vi "函数类型1测试.vi"() -> ()   [LabVIEW 2010]
uses:
  全局量/试验配置信息.vi
panel:
  out "D_IN_1":string[][](table) caption="表格"
  in  "加载文件名称":string
  out "配置文件路径":path
  out "配置文件目录":path
  in  "同步_1":i32
  in  "数组_反馈值":dbl[][](array[numeric])
  in  "第几个数据":i32
  in  "第几组数据":i32
  in  "数组_设定值":dbl[][](array[numeric])
  in  "数组_选择":bool[](array[boolean])
  out "light_32":bool
  out "light_31":bool
  out "light_30":bool
  out "light_29":bool
  out "light_28":bool
  out "light_27":bool
  out "light_26":bool
  out "light_25":bool
  out "light_24":bool
  out "light_23":bool
  out "light_22":bool
  out "light_21":bool
  out "light_20":bool
  out "light_19":bool
  out "light_18":bool
  out "light_17":bool
  out "Analog_back":string[][](table) caption="表格"
  in  "A_32":bool
  in  "A_31":bool
  in  "A_30":bool
  in  "A_29":bool
  in  "A_28":bool
  in  "A_27":bool
  in  "A_26":bool
  in  "A_25":bool
  in  "A_24":bool
  in  "A_23":bool
  in  "A_22":bool
  in  "A_21":bool
  in  "A_20":bool
  in  "A_19":bool
  in  "A_18":bool
  in  "A_17":bool
  out "合格？":bool[][](array[boolean])
  out "测试结论":string
  out "light_16":bool
  out "light_15":bool
  out "light_14":bool
  out "light_13":bool
  out "light_12":bool
  out "light_11":bool
  out "light_10":bool
  out "light_9":bool
  out "light_8":bool
  out "light_7":bool
  out "light_6":bool
  out "light_5":bool
  out "light_4":bool
  out "light_3":bool
  out "light_2":bool
  out "light_1":bool
  out "退出？":bool
  in  "btn_反选":bool
  in  "btn_全选":bool
  in  "A_16":bool
  in  "A_15":bool
  in  "A_14":bool
  in  "A_13":bool
  in  "A_12":bool
  in  "A_11":bool
  in  "A_10":bool
  in  "A_9":bool
  in  "A_8":bool
  in  "A_7":bool
  in  "A_6":bool
  in  "A_5":bool
  in  "A_4":bool
  in  "A_3":bool
  in  "A_2":bool
  in  "A_1":bool
  in  "btn_取消":bool
  in  "btn_开始测试":bool
  in  "Analog_IN":string[][](table) caption="表格"
  out "Analog_WC":string[][](table) caption="表格"
  # "模拟量选择及输入值（V）"
  # "模拟量反馈值（V）"
  # "模拟量误差值（%）"
  # "测试结论："
  # "从0开始"
  # "从1开始,第0列没有使用"
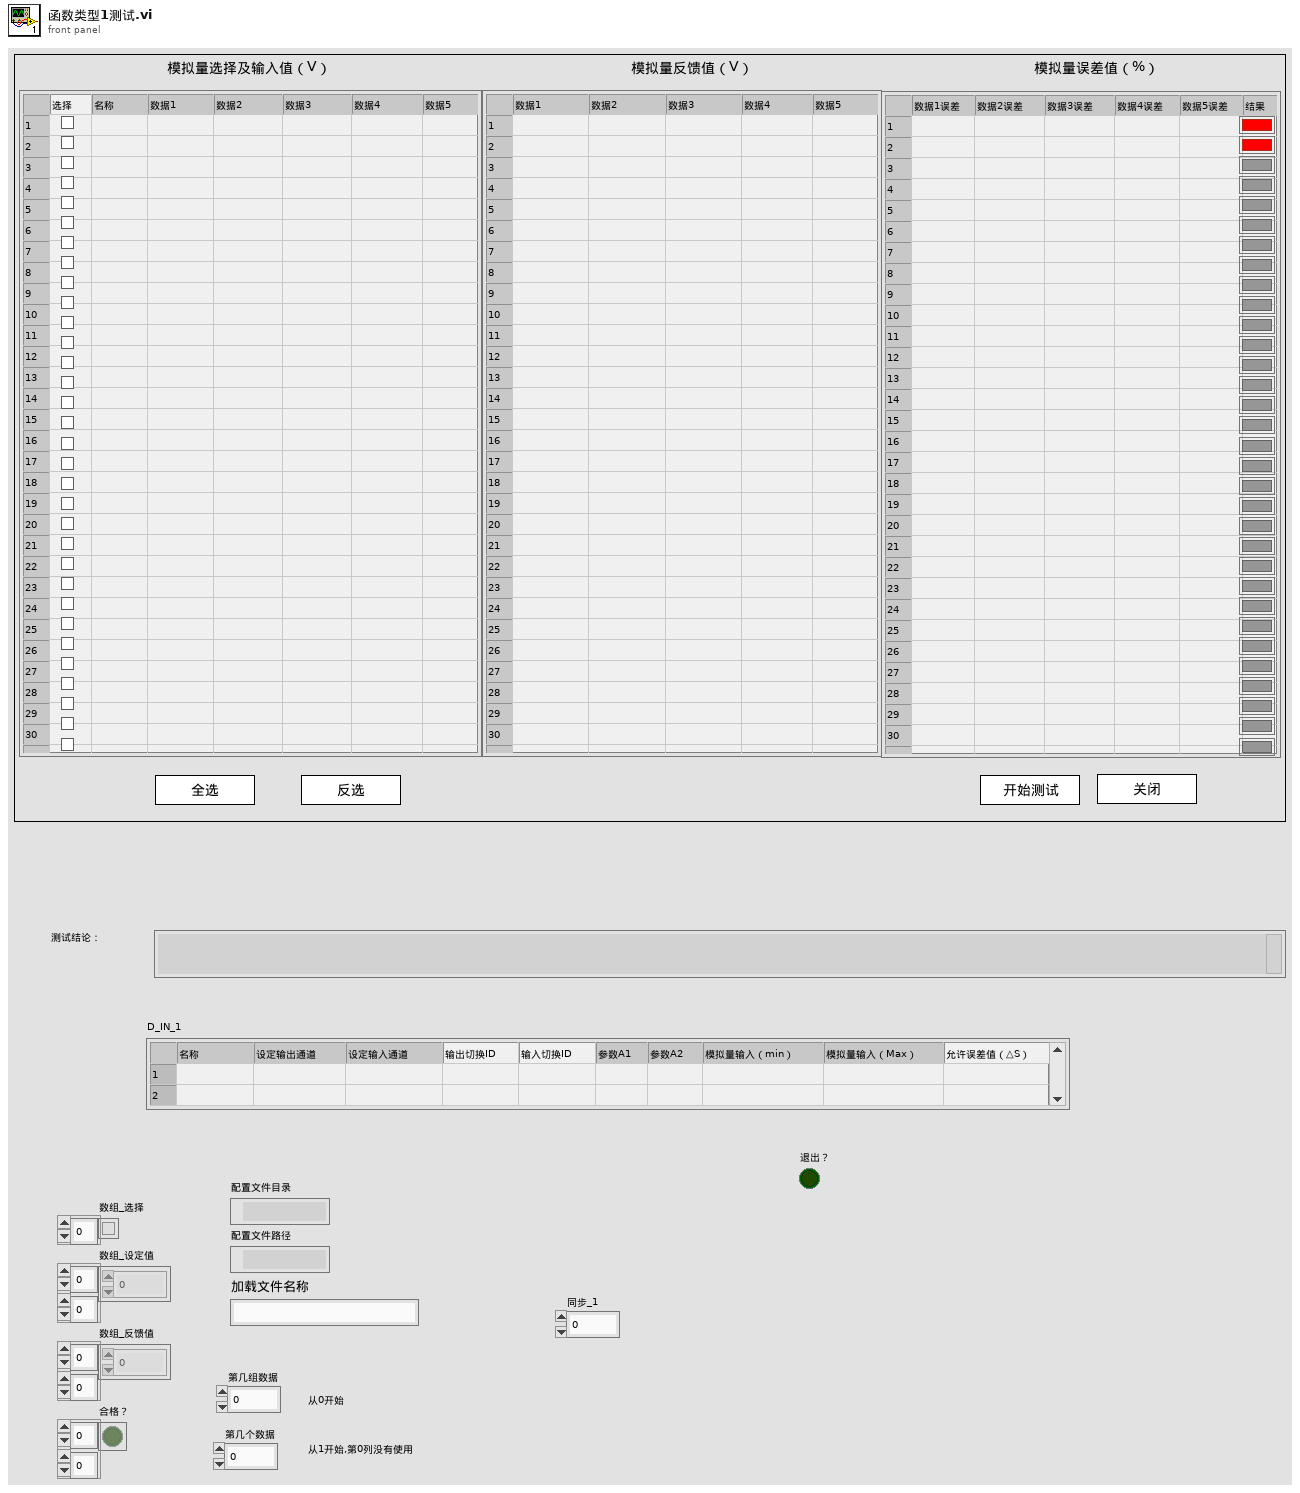
[diagram p1: front panel]
types:
  T1 = enum8{"Enabled", "Disabled", "Disabled and Grayed Out"}
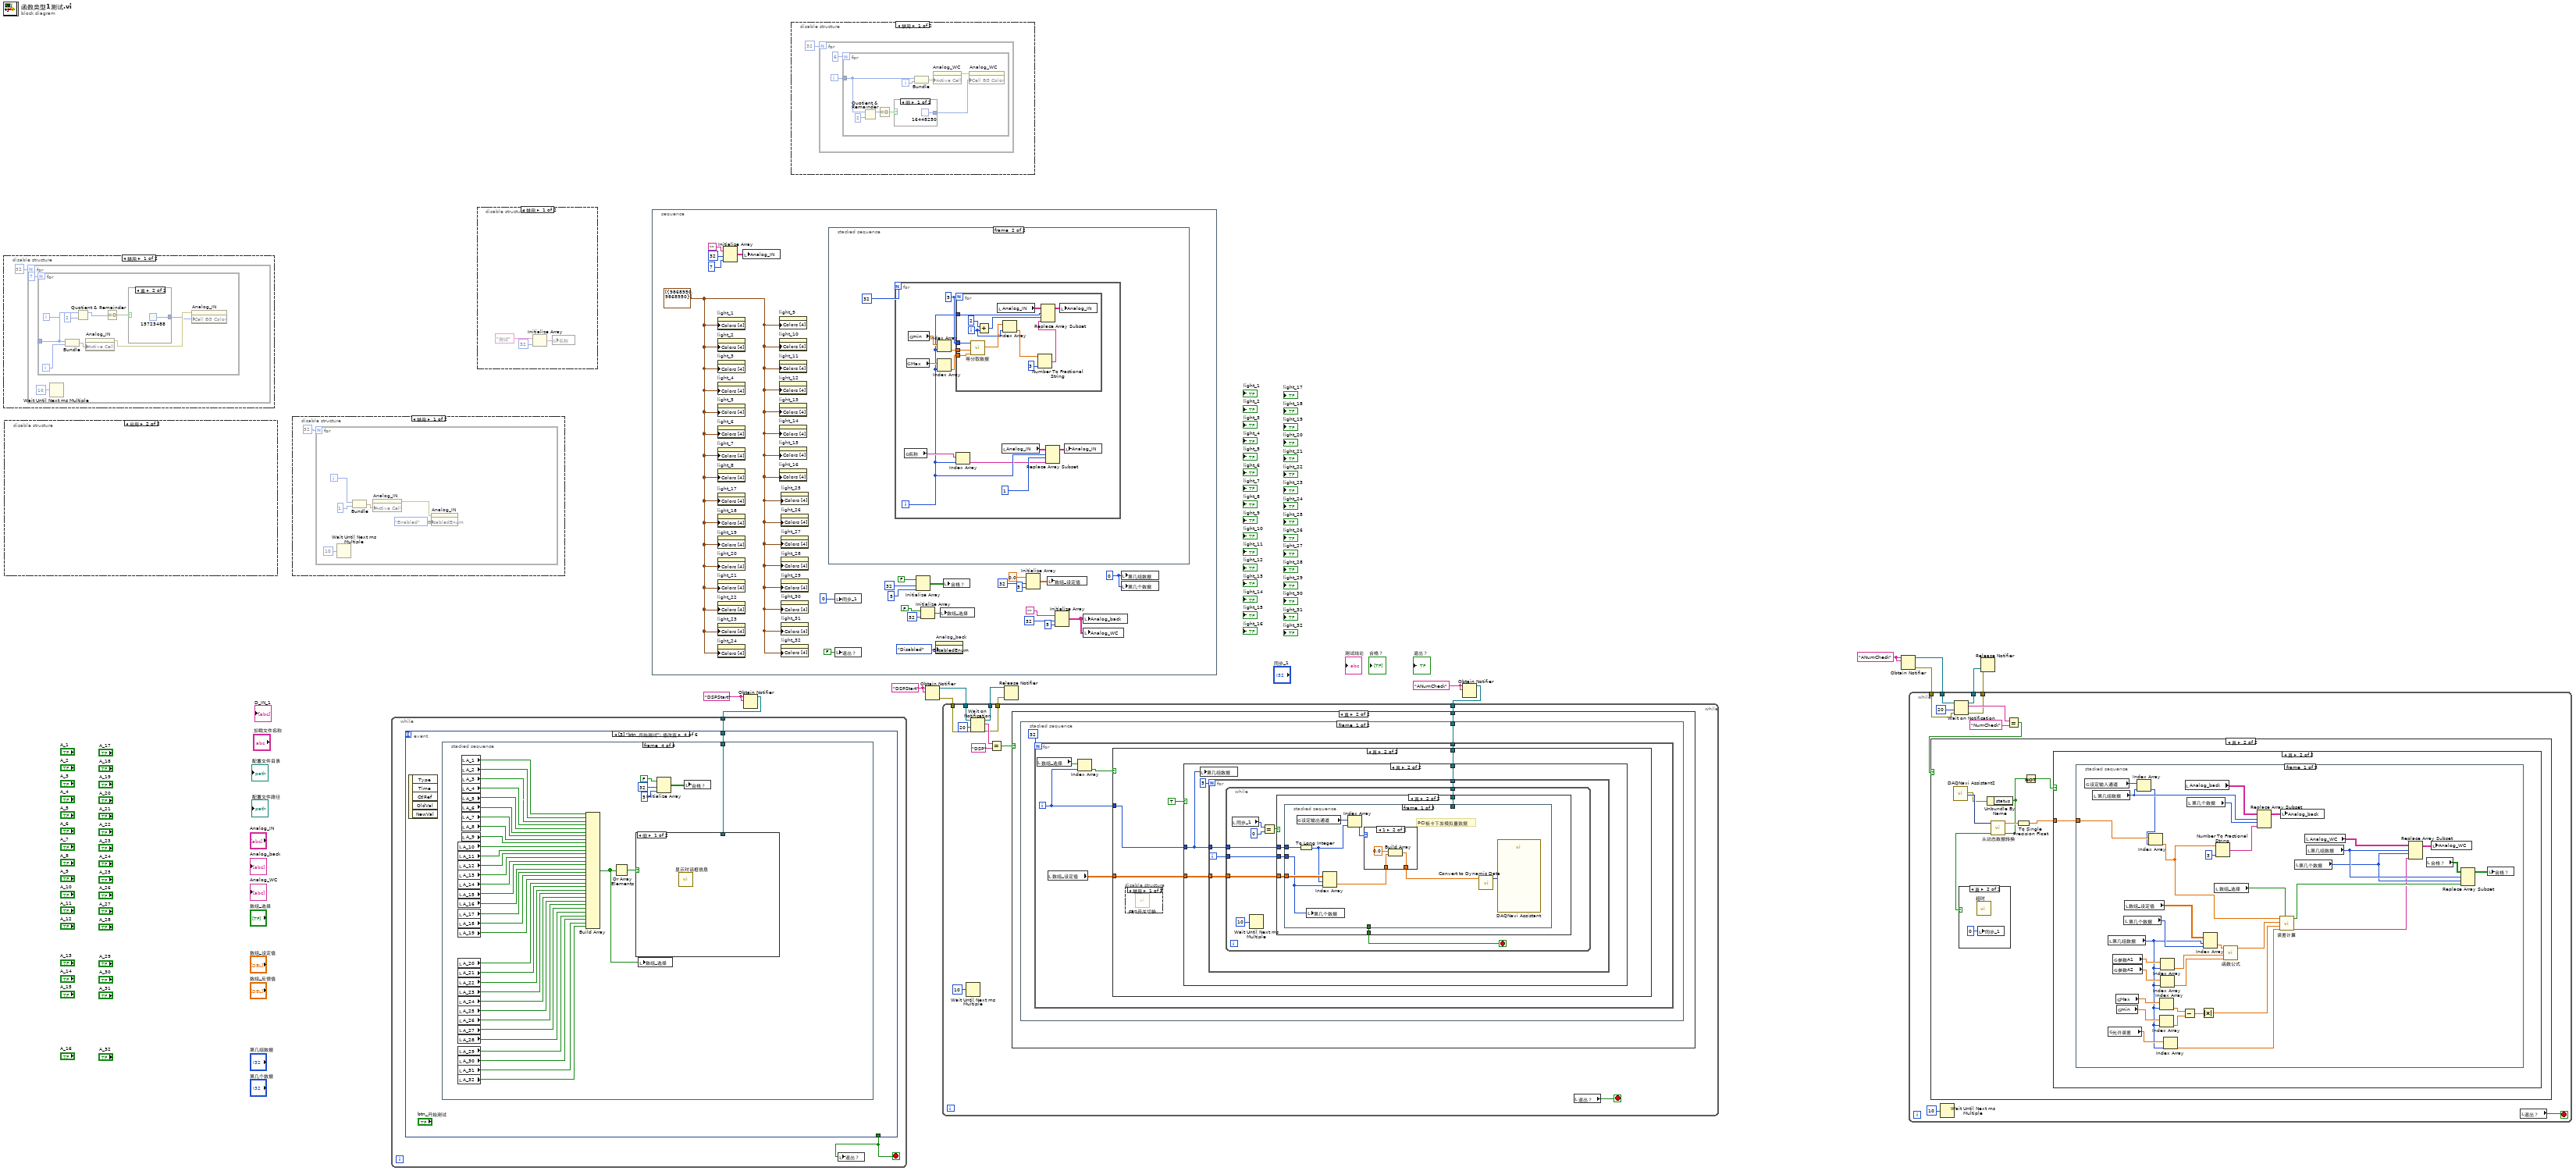
[diagram p0: block diagram]
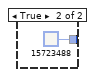
[diagram p2: hidden frame]
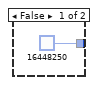
[diagram p5: hidden frame]
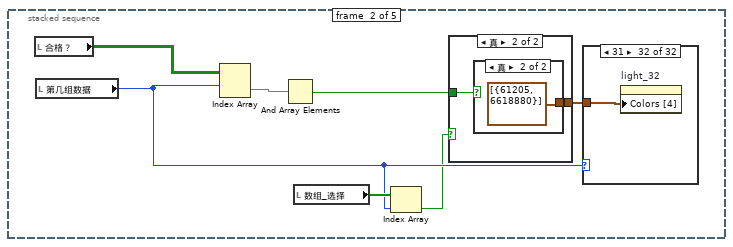
[diagram p10: hidden frame]
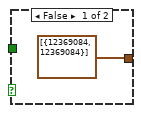
[diagram p11: hidden frame]
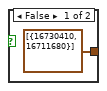
[diagram p12: hidden frame]
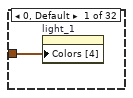
[diagram p13: hidden frame]
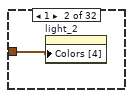
[diagram p14: hidden frame]
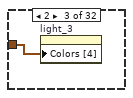
[diagram p15: hidden frame]
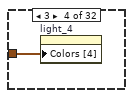
[diagram p16: hidden frame]
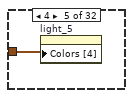
[diagram p17: hidden frame]
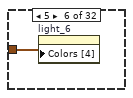
[diagram p18: hidden frame]
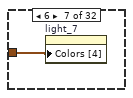
[diagram p19: hidden frame]
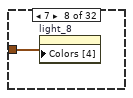
[diagram p20: hidden frame]
diagram:
  w2 = "ANumCheck" ("名称（未命名）")
  w4 = "DSPStart" ("名称（未命名）")
  w9 = "ANumCheck" ("名称（未命名）")
  w12 = "DSPStart" ("名称（未命名）")
  n1 = disable-structure shown="禁用" {
    frame Disabled {
      n2 = for {
        N: 32 -> [_]
        i -> [w17]
        n3 = for {
          N: 7 -> [_]
          tunnel: w17 -> [w25]
          i -> [w19]
          n4 = Bundle(w25, w19) -> (w22:cluster{i32, i32})  [unwired: 1 in]
          n5 = Quotient & Remainder(x=w25, y=2) -> (x-y*floor(x/y)=w23:i32)  [unwired: 1 out]
          n6 = property on="Analog_IN" class="Tbl (严格)"("Active Cell"=w22) -> (error out=w21:errorcluster)  [unwired: 2 in, 1 out]
          n7 = Equal To 0?(x=w23) -> (x = 0?=w26:bool)
          n8 = case shown="真" w26 {
            tunnel: [u32 16448250 u32 15723488] -> w20
            frame False {
            }
            frame True {
            }
          }
          n9 = property on="Analog_IN" class="Tbl (严格)"(error in=w21, "Cell BG Color"=w20) -> ()  [unwired: 1 in, 2 out]
        }
        n10 = Wait Until Next ms Multiple(millisecond multiple=u32 10 ("毫秒倍数")) -> ()  [unwired: 1 out]
      }
    }
    frame Enabled {
    }
  }
  n11 = disable-structure shown="启用" {
    frame Disabled {
      n12 = for {
        N: 32 -> [_]
        i -> [w30]
        n13 = for {
          N: 7 -> [_]
          tunnel: w30 -> [w33]
          i -> [w34]
          n14 = Bundle(w33, w34) -> (w37:cluster{i32, i32})  [unwired: 1 in]
          n15 = property on="Analog_IN" class="Tbl (严格)"("Active Cell"=w37) -> (error out=w35:errorcluster)  [unwired: 2 in, 1 out]
          n16 = property on="Analog_IN" class="Tbl (严格)"(error in=w35, "Justify"=enum16{"Left", "Center", "Right"}."Left" ("活动单元格:单元格对齐")) -> ()  [unwired: 1 in, 2 out]
        }
        n17 = Wait Until Next ms Multiple(millisecond multiple=u32 10 ("毫秒倍数")) -> ()  [unwired: 1 out]
      }
    }
    frame Enabled {
    }
  }
  n18 = disable-structure shown="禁用" {
    frame Disabled {
      n19 = for {
        N: 32 -> [_]
        i -> [w43]
        n20 = Wait Until Next ms Multiple(millisecond multiple=u32 10 ("毫秒倍数")) -> ()  [unwired: 1 out]
        n21 = Bundle(w43, 1) -> (w42:cluster{i32, i32})  [unwired: 1 in]
        n22 = property on="Analog_IN" class="Tbl (严格)"("Active Cell"=w42) -> (error out=w39:errorcluster)  [unwired: 2 in, 1 out]
        n23 = property on="Analog_IN" class="Tbl (严格)"(error in=w39, "DisabledEnum"=T1."Enabled" ("禁用")) -> ()  [unwired: 1 in, 2 out]
      }
    }
    frame Enabled {
    }
  }
  n24 = disable-structure shown="禁用" {
    frame Disabled {
      n25 = Initialize Array("测试", 32 ("维数大小")) -> (w46:string[])
      n26 = global write "试验配置信息.vi" "名称"(w46) -> ()
    }
    frame Enabled {
    }
  }
  n27 = stacked-sequence {
    frame #0 {
      w52 = 0 ("第几组数据")
      w67 = cluster{u32, u32}[] [{9868950, 9868950}]
      n28 = property on="light_1" class="Bool (严格)"("Colors [4]"=w67) -> ()  [unwired: 2 in, 2 out]
      n29 = property on="light_2" class="Bool (严格)"("Colors [4]"=w67) -> ()  [unwired: 2 in, 2 out]
      n30 = property on="light_3" class="Bool (严格)"("Colors [4]"=w67) -> ()  [unwired: 2 in, 2 out]
      n31 = property on="light_4" class="Bool (严格)"("Colors [4]"=w67) -> ()  [unwired: 2 in, 2 out]
      n32 = property on="light_5" class="Bool (严格)"("Colors [4]"=w67) -> ()  [unwired: 2 in, 2 out]
      n33 = property on="light_6" class="Bool (严格)"("Colors [4]"=w67) -> ()  [unwired: 2 in, 2 out]
      n34 = property on="light_7" class="Bool (严格)"("Colors [4]"=w67) -> ()  [unwired: 2 in, 2 out]
      n35 = property on="light_8" class="Bool (严格)"("Colors [4]"=w67) -> ()  [unwired: 2 in, 2 out]
      n36 = property on="light_17" class="Bool (严格)"("Colors [4]"=w67) -> ()  [unwired: 2 in, 2 out]
      n37 = property on="light_18" class="Bool (严格)"("Colors [4]"=w67) -> ()  [unwired: 2 in, 2 out]
      n38 = property on="light_19" class="Bool (严格)"("Colors [4]"=w67) -> ()  [unwired: 2 in, 2 out]
      n39 = property on="light_20" class="Bool (严格)"("Colors [4]"=w67) -> ()  [unwired: 2 in, 2 out]
      n40 = property on="light_21" class="Bool (严格)"("Colors [4]"=w67) -> ()  [unwired: 2 in, 2 out]
      n41 = property on="light_22" class="Bool (严格)"("Colors [4]"=w67) -> ()  [unwired: 2 in, 2 out]
      n42 = property on="light_23" class="Bool (严格)"("Colors [4]"=w67) -> ()  [unwired: 2 in, 2 out]
      n43 = property on="light_24" class="Bool (严格)"("Colors [4]"=w67) -> ()  [unwired: 2 in, 2 out]
      n44 = Initialize Array("", 32 ("维数大小"), 7 ("维数大小")) -> (w51:string[][])
      n45 = local write "Analog_IN"(w51) -> ()
      n46 = property on="light_9" class="Bool (严格)"("Colors [4]"=w67) -> ()  [unwired: 2 in, 2 out]
      n47 = property on="light_10" class="Bool (严格)"("Colors [4]"=w67) -> ()  [unwired: 2 in, 2 out]
      n48 = property on="light_11" class="Bool (严格)"("Colors [4]"=w67) -> ()  [unwired: 2 in, 2 out]
      n49 = property on="light_12" class="Bool (严格)"("Colors [4]"=w67) -> ()  [unwired: 2 in, 2 out]
      n50 = property on="light_13" class="Bool (严格)"("Colors [4]"=w67) -> ()  [unwired: 2 in, 2 out]
      n51 = property on="light_14" class="Bool (严格)"("Colors [4]"=w67) -> ()  [unwired: 2 in, 2 out]
      n52 = property on="light_15" class="Bool (严格)"("Colors [4]"=w67) -> ()  [unwired: 2 in, 2 out]
      n53 = property on="light_16" class="Bool (严格)"("Colors [4]"=w67) -> ()  [unwired: 2 in, 2 out]
      n54 = property on="light_25" class="Bool (严格)"("Colors [4]"=w67) -> ()  [unwired: 2 in, 2 out]
      n55 = property on="light_26" class="Bool (严格)"("Colors [4]"=w67) -> ()  [unwired: 2 in, 2 out]
      n56 = property on="light_27" class="Bool (严格)"("Colors [4]"=w67) -> ()  [unwired: 2 in, 2 out]
      n57 = property on="light_28" class="Bool (严格)"("Colors [4]"=w67) -> ()  [unwired: 2 in, 2 out]
      n58 = property on="light_29" class="Bool (严格)"("Colors [4]"=w67) -> ()  [unwired: 2 in, 2 out]
      n59 = property on="light_30" class="Bool (严格)"("Colors [4]"=w67) -> ()  [unwired: 2 in, 2 out]
      n60 = property on="light_31" class="Bool (严格)"("Colors [4]"=w67) -> ()  [unwired: 2 in, 2 out]
      n61 = property on="light_32" class="Bool (严格)"("Colors [4]"=w67) -> ()  [unwired: 2 in, 2 out]
      n62 = stacked-sequence {
        frame #0 {
          n63 = for {
            N: 32 ("维数大小") -> [_]
            tunnel: [w112] -> w76 mode=indexing
            tunnel: [w108] -> w75 mode=indexing
            tunnel: [w106] -> w74 mode=indexing
            tunnel: [w103] -> w73 mode=indexing
            tunnel: [w100] -> w72 mode=indexing
            tunnel: [w97] -> w78 mode=indexing
            tunnel: [w94] -> w79 mode=indexing
            tunnel: [w91] -> w80 mode=indexing
            tunnel: [w88] -> w81 mode=indexing
            tunnel: [w84] -> w82 mode=indexing
            i -> [w86]
            n64 = global read "试验配置信息.vi" "D_IN_1"() -> (w83:string[][])
            n65 = Index Array(array=w83, index (row)=w86, index (col)=0 ("禁用的索引 (列)")) -> (element=w112:string)
            n66 = Index Array(array=w83, index (row)=w86, index (col)=2 ("禁用的索引 (列)")) -> (element=w102:string)
            n67 = Index Array(array=w83, index (row)=w86, index (col)=3 ("禁用的索引 (列)")) -> (element=w98:string)
            n68 = Index Array(array=w83, index (row)=w86, index (col)=4 ("禁用的索引 (列)")) -> (element=w96:string)
            n69 = Index Array(array=w83, index (row)=w86, index (col)=5 ("禁用的索引 (列)")) -> (element=w93:string)
            n70 = Index Array(array=w83, index (row)=w86, index (col)=9 ("禁用的索引 (列)")) -> (element=w85:string)
            n71 = Index Array(array=w83, index (row)=w86, index (col)=1 ("禁用的索引 (列)")) -> (element=w105:string)
            n72 = Index Array(array=w83, index (row)=w86, index (col)=6 ("禁用的索引 (列)")) -> (element=w89:string)
            n73 = Index Array(array=w83, index (row)=w86, index (col)=7 ("禁用的索引 (列)")) -> (element=w109:string)
            n74 = Index Array(array=w83, index (row)=w86, index (col)=8 ("禁用的索引 (列)")) -> (element=w107:string)
            n75 = Decimal String To Number(string=w102) -> (number=w100:i32)  [unwired: 2 in, 1 out]
            n76 = Decimal String To Number(string=w98) -> (number=w97:i32)  [unwired: 2 in, 1 out]
            n77 = Decimal String To Number(string=w96) -> (number=w94:i32)  [unwired: 2 in, 1 out]
            n78 = Decimal String To Number(string=w105) -> (number=w103:i32)  [unwired: 2 in, 1 out]
            n79 = Fract/Exp String To Number(string=w93) -> (number=w91:dbl)  [unwired: 3 in, 1 out]
            n80 = Fract/Exp String To Number(string=w85) -> (number=w84:dbl)  [unwired: 3 in, 1 out]
            n81 = Fract/Exp String To Number(string=w89) -> (number=w88:dbl)  [unwired: 3 in, 1 out]
            n82 = Fract/Exp String To Number(string=w109) -> (number=w108:dbl)  [unwired: 3 in, 1 out]
            n83 = Fract/Exp String To Number(string=w107) -> (number=w106:dbl)  [unwired: 3 in, 1 out]
          }
          n84 = global write "试验配置信息.vi" "名称"(w76) -> ()
          n85 = global write "试验配置信息.vi" "设定输入通道"(w72) -> ()
          n86 = global write "试验配置信息.vi" "输出切换ID"(w78) -> ()
          n87 = global write "试验配置信息.vi" "输入切换ID"(w79) -> ()
          n88 = global write "试验配置信息.vi" "参数A1"(w80) -> ()
          n89 = global write "试验配置信息.vi" "允许误差"(w82) -> ()
          n90 = global write "试验配置信息.vi" "设定输出通道"(w73) -> ()
          n91 = global write "试验配置信息.vi" "参数A2"(w81) -> ()
          n92 = global write "试验配置信息.vi" "min"(w75) -> ()
          n93 = global write "试验配置信息.vi" "Max"(w74) -> ()
        }
        frame #1 {
          n94 = for {
            N: 32 -> [_]
            i -> [w117]
            w121 = 5 ("num")
            n95 = global read "试验配置信息.vi" "名称"() -> (w120:string[])
            n96 = global read "试验配置信息.vi" "Max"() -> (w124:dbl[])
            n97 = global read "试验配置信息.vi" "min"() -> (w125:dbl[])
            n98 = Index Array(array=w125, index=w117) -> (element=w123:dbl)
            n99 = Index Array(array=w124, index=w117) -> (element=w122:dbl)
            n100 = for {
              N: w121 -> [_]
              tunnel: w117 -> [w136]
              tunnel: w123 -> [w133]
              tunnel: w122 -> [w132]
              tunnel: w121 -> [w131]
              i -> [w129]
              n101 = call "等分取数据.vi"("Max"=w132, "MIN"=w133, "num"=w131) -> ("数据点"=w130:dbl[])  [unwired: 5 in]
              n102 = Add(x=2, y=w129) -> (x+y=w134:i32)
              n103 = local read "Analog_IN"() -> (w138:string[][])
              n104 = Index Array(array=w130, index=w129) -> (element=w127:dbl)
              n105 = Number To Fractional String(number=w127, precision (6)=i16 3 ("精度(6)")) -> (F-format string=w128:string)  [unwired: 2 in]
              n106 = Replace Array Subset(array=w138, new element=w128, index (row)=w136, index (col)=w134) -> (w137:string[][])
              n107 = local write "Analog_IN"(w137) -> ()
            }
            n108 = Index Array(array=w120, index=w117) -> (element=w115:string)
            n109 = local read "Analog_IN"() -> (w118:string[][])
            n110 = Replace Array Subset(array=w118, new element=w115, index (row)=w117, index (col)=1) -> (w119:string[][])
            n111 = local write "Analog_IN"(w119) -> ()
          }
        }
      }
      n112 = local write "同步_1"(0 ("同步_2")) -> ()
      n113 = local write "退出？"(FALSE ("退出？")) -> ()
      n114 = Initialize Array(FALSE, 32 ("维数大小"), 5 ("维数大小")) -> (w68:bool[][])
      n115 = Initialize Array(FALSE, 32 ("维数大小")) -> (w56:bool[])
      n116 = property on="Analog_back" class="Tbl (严格)"("DisabledEnum"=T1."Disabled" ("禁用")) -> ()  [unwired: 2 in, 2 out]
      n117 = local write "数组_选择"(w56) -> ()
      n118 = local write "合格？"(w68) -> ()
      n119 = Initialize Array(0.0, 32 ("维数大小"), 5 ("维数大小")) -> (w59:dbl[][])
      n120 = local write "数组_设定值"(w59) -> ()
      n121 = Initialize Array("", 32 ("维数大小"), 5 ("维数大小")) -> (w63:string[][])
      n122 = local write "Analog_back"(w63) -> ()
      n123 = local write "Analog_WC"(w63) -> ()
      n124 = local write "第几组数据"(w52) -> ()
      n125 = local write "第几个数据"(w52) -> ()
    }
  }
  n126 = Obtain Notifier(name (unnamed)=w4, notification data type=w4) -> (notifier out=w3:refnum<notifier>)  [unwired: 2 in, 2 out]
  n127 = while {
    tunnel: w3 -> [w139]
    stop <- w140 stop-if-true
    n128 = event shown="[3] \"btn_开始测试\": 值改变" {
      selector: _ -> [_ _ _ _ _ _]
      dyn-events: _ -> [_ _ _ _ _ _]
      timeout: _ -> [_ _ _ _ _ _]
      tunnel: [_ TRUE TRUE _ _ _] -> w140
      tunnel: w139 -> [_ _ _ w143 _ _]
      event Timeout {
        n129 = event-data() -> ()  [unwired: 1 in, 2 out]
      }
      event Panel Close {
        n130 = event-data() -> ()  [unwired: 1 in, 3 out]
      }
      event "btn_取消": Value Change {
        n131 = event-data() -> ()  [unwired: 1 in, 5 out]
      }
      event "btn_开始测试": Value Change {
        n132 = event-data() -> ()  [unwired: 1 in, 5 out]
        n133 = stacked-sequence {
          tunnel: w143 -> [_ _ _ w226]
          frame #0 {
            w149 = 0 ("第几组数据")
            # "测试期间不准退出防止程序卡死"
            n134 = local read "Analog_IN"() -> (w155:string[][])
            n135 = Delete From Array(array=w155, length=1 ("长度"), index (col)=0 ("禁用的索引 (列)")) -> (array with subset deleted=w147:string[][])  [unwired: 1 in, 1 out]
            n136 = Delete From Array(array=w147, length=1 ("长度"), index (col)=0 ("禁用的索引 (列)")) -> (array with subset deleted=w145:string[][])  [unwired: 1 in, 1 out]
            n137 = for {
              N: 32 -> [_]
              tunnel: w145 -> [w158] mode=indexing
              tunnel: [w157] -> w154 mode=indexing
              n138 = for {
                N: 5 -> [_]
                tunnel: w158 -> [w160] mode=indexing
                tunnel: [w159] -> w157 mode=indexing
                n139 = Fract/Exp String To Number(string=w160) -> (number=w159:dbl)  [unwired: 3 in, 1 out]
              }
            }
            n140 = local write "第几组数据"(w149) -> ()
            n141 = local write "第几个数据"(w149) -> ()
            n142 = local write "同步_1"(0 ("同步_2")) -> ()
            n143 = property on="btn_取消" class="Bool"("DisabledEnum"=T1."Disabled and Grayed Out" ("禁用")) -> ()  [unwired: 2 in, 2 out]
            n144 = local write "数组_设定值"(w154) -> ()
          }
          frame #1 {
            n145 = local read "Analog_back"() -> (w163:string[][])
            n146 = local read "Analog_WC"() -> (w162:string[][])
            n147 = for {
              tunnel: w162 -> [w199] mode=indexing
              i -> [w198]
              n148 = for {
                tunnel: w199 -> [_] mode=indexing
                tunnel: w198 -> [w203]
                i -> [w202]
                n149 = local read "Analog_WC"() -> (w204:string[][])
                n150 = Replace Array Subset(array=w204, new element="", index (row)=w203, index (col)=w202) -> (w200:string[][])
                n151 = local write "Analog_WC"(w200) -> ()
              }
            }
            n152 = for {
              tunnel: w163 -> [w206] mode=indexing
              i -> [w205]
              n153 = for {
                tunnel: w206 -> [_] mode=indexing
                tunnel: w205 -> [w210]
                i -> [w209]
                n154 = local read "Analog_back"() -> (w211:string[][])
                n155 = Replace Array Subset(array=w211, new element="", index (row)=w210, index (col)=w209) -> (w207:string[][])
                n156 = local write "Analog_back"(w207) -> ()
              }
            }
            n157 = for {
              N: 32 -> [_]
              i -> [w165]
              n158 = case shown="31" w165 {
                tunnel: cluster{u32, u32}[] [{9868950, 9868950}] -> [w166 w167 w168 w169 w170 w171 w172 w173 w174 w175 w176 w177 w178 w179 w180 w181 w182 w183 w184 w185 w186 w187 w188 w189 w190 w191 w192 w193 w194 w195 w196 w197]
                frame 0, Default {
                  n159 = property on="light_1" class="Bool (严格)"("Colors [4]"=w166) -> ()  [unwired: 2 in, 2 out]
                }
                frame 1 {
                  n160 = property on="light_2" class="Bool (严格)"("Colors [4]"=w167) -> ()  [unwired: 2 in, 2 out]
                }
                frame 2 {
                  n161 = property on="light_3" class="Bool (严格)"("Colors [4]"=w168) -> ()  [unwired: 2 in, 2 out]
                }
                frame 3 {
                  n162 = property on="light_4" class="Bool (严格)"("Colors [4]"=w169) -> ()  [unwired: 2 in, 2 out]
                }
                frame 4 {
                  n163 = property on="light_5" class="Bool (严格)"("Colors [4]"=w170) -> ()  [unwired: 2 in, 2 out]
                }
                frame 5 {
                  n164 = property on="light_6" class="Bool (严格)"("Colors [4]"=w171) -> ()  [unwired: 2 in, 2 out]
                }
                frame 6 {
                  n165 = property on="light_7" class="Bool (严格)"("Colors [4]"=w172) -> ()  [unwired: 2 in, 2 out]
                }
                frame 7 {
                  n166 = property on="light_8" class="Bool (严格)"("Colors [4]"=w173) -> ()  [unwired: 2 in, 2 out]
                }
                frame 8 {
                  n167 = property on="light_9" class="Bool (严格)"("Colors [4]"=w174) -> ()  [unwired: 2 in, 2 out]
                }
                frame 9 {
                  n168 = property on="light_10" class="Bool (严格)"("Colors [4]"=w175) -> ()  [unwired: 2 in, 2 out]
                }
                frame 10 {
                  n169 = property on="light_11" class="Bool (严格)"("Colors [4]"=w176) -> ()  [unwired: 2 in, 2 out]
                }
                frame 11 {
                  n170 = property on="light_12" class="Bool (严格)"("Colors [4]"=w177) -> ()  [unwired: 2 in, 2 out]
                }
                frame 12 {
                  n171 = property on="light_13" class="Bool (严格)"("Colors [4]"=w178) -> ()  [unwired: 2 in, 2 out]
                }
                frame 13 {
                  n172 = property on="light_14" class="Bool (严格)"("Colors [4]"=w179) -> ()  [unwired: 2 in, 2 out]
                }
                frame 14 {
                  n173 = property on="light_15" class="Bool (严格)"("Colors [4]"=w180) -> ()  [unwired: 2 in, 2 out]
                }
                frame 15 {
                  n174 = property on="light_16" class="Bool (严格)"("Colors [4]"=w181) -> ()  [unwired: 2 in, 2 out]
                }
                frame 16 {
                  n175 = property on="light_17" class="Bool (严格)"("Colors [4]"=w182) -> ()  [unwired: 2 in, 2 out]
                }
                frame 17 {
                  n176 = property on="light_18" class="Bool (严格)"("Colors [4]"=w183) -> ()  [unwired: 2 in, 2 out]
                }
                frame 18 {
                  n177 = property on="light_19" class="Bool (严格)"("Colors [4]"=w184) -> ()  [unwired: 2 in, 2 out]
                }
                frame 19 {
                  n178 = property on="light_20" class="Bool (严格)"("Colors [4]"=w185) -> ()  [unwired: 2 in, 2 out]
                }
                frame 20 {
                  n179 = property on="light_21" class="Bool (严格)"("Colors [4]"=w186) -> ()  [unwired: 2 in, 2 out]
                }
                frame 21 {
                  n180 = property on="light_22" class="Bool (严格)"("Colors [4]"=w187) -> ()  [unwired: 2 in, 2 out]
                }
                frame 22 {
                  n181 = property on="light_23" class="Bool (严格)"("Colors [4]"=w188) -> ()  [unwired: 2 in, 2 out]
                }
                frame 23 {
                  n182 = property on="light_24" class="Bool (严格)"("Colors [4]"=w189) -> ()  [unwired: 2 in, 2 out]
                }
                frame 24 {
                  n183 = property on="light_25" class="Bool (严格)"("Colors [4]"=w190) -> ()  [unwired: 2 in, 2 out]
                }
                frame 25 {
                  n184 = property on="light_26" class="Bool (严格)"("Colors [4]"=w191) -> ()  [unwired: 2 in, 2 out]
                }
                frame 26 {
                  n185 = property on="light_27" class="Bool (严格)"("Colors [4]"=w192) -> ()  [unwired: 2 in, 2 out]
                }
                frame 27 {
                  n186 = property on="light_28" class="Bool (严格)"("Colors [4]"=w193) -> ()  [unwired: 2 in, 2 out]
                }
                frame 28 {
                  n187 = property on="light_29" class="Bool (严格)"("Colors [4]"=w194) -> ()  [unwired: 2 in, 2 out]
                }
                frame 29 {
                  n188 = property on="light_30" class="Bool (严格)"("Colors [4]"=w195) -> ()  [unwired: 2 in, 2 out]
                }
                frame 30 {
                  n189 = property on="light_31" class="Bool (严格)"("Colors [4]"=w196) -> ()  [unwired: 2 in, 2 out]
                }
                frame 31 {
                  n190 = property on="light_32" class="Bool (严格)"("Colors [4]"=w197) -> ()  [unwired: 2 in, 2 out]
                }
              }
            }
          }
          frame #2 {
            n191 = for {
              N: 32 -> [_]
              i -> [w214]
              n192 = disable-structure shown="禁用" {
                frame Disabled {
                  n193 = Wait Until Next ms Multiple(millisecond multiple=u32 10 ("毫秒倍数")) -> ()  [unwired: 1 out]
                }
                frame Enabled {
                }
              }
              n194 = for {
                N: 6 -> [_]
                tunnel: w214 -> [w222]
                i -> [w219]
                n195 = Quotient & Remainder(x=w222, y=2) -> (x-y*floor(x/y)=w220:i32)  [unwired: 1 out]
                n196 = Equal To 0?(x=w220) -> (x = 0?=w223:bool)
                n197 = case shown="假" w223 {
                  tunnel: [u32 16448250 u32 15723488] -> w216
                  frame False {
                  }
                  frame True {
                  }
                }
                n198 = Bundle(w222, w219) -> (w218:cluster{i32, i32})  [unwired: 1 in]
                n199 = property on="Analog_WC" class="Tbl (严格)"("Active Cell"=w218) -> (error out=w217:errorcluster)  [unwired: 2 in, 1 out]
                n200 = property on="Analog_WC" class="Tbl (严格)"(error in=w217, "Cell BG Color"=w216) -> ()  [unwired: 1 in, 2 out]
              }
            }
          }
          frame #3 {
            n201 = local read "A_10"() -> (w255:bool)
            n202 = local read "A_11"() -> (w254:bool)
            n203 = local read "A_12"() -> (w253:bool)
            n204 = local read "A_13"() -> (w252:bool)
            n205 = local read "A_14"() -> (w251:bool)
            n206 = local read "A_15"() -> (w250:bool)
            n207 = local read "A_16"() -> (w249:bool)
            n208 = local read "A_17"() -> (w248:bool)
            n209 = local read "A_18"() -> (w247:bool)
            n210 = local read "A_19"() -> (w246:bool)
            n211 = local read "A_20"() -> (w245:bool)
            n212 = local read "A_21"() -> (w244:bool)
            n213 = local read "A_22"() -> (w243:bool)
            n214 = local read "A_23"() -> (w242:bool)
            n215 = local read "A_24"() -> (w241:bool)
            n216 = local read "A_25"() -> (w240:bool)
            n217 = local read "A_26"() -> (w239:bool)
            n218 = local read "A_27"() -> (w238:bool)
            n219 = local read "A_28"() -> (w237:bool)
            n220 = local read "A_29"() -> (w236:bool)
            n221 = local read "A_30"() -> (w235:bool)
            n222 = local read "A_31"() -> (w234:bool)
            n223 = local read "A_32"() -> (w233:bool)
            n224 = local read "A_1"() -> (w264:bool)
            n225 = local read "A_2"() -> (w263:bool)
            n226 = local read "A_3"() -> (w262:bool)
            n227 = local read "A_4"() -> (w261:bool)
            n228 = local read "A_5"() -> (w260:bool)
            n229 = local read "A_6"() -> (w259:bool)
            n230 = local read "A_7"() -> (w258:bool)
            n231 = local read "A_8"() -> (w257:bool)
            n232 = local read "A_9"() -> (w256:bool)
            n233 = Build Array(w264, w263, w262, w261, w260, w259, w258, w257, w256, w255, w254, w253, w252, w251, w250, w249, w248, w247, w246, w245, w244, w243, w242, w241, w240, w239, w238, w237, w236, w235, w234, w233) -> (w227:bool[])
            n234 = Or Array Elements(Boolean array=w227) -> (logical OR=w232:bool)
            n235 = case shown="假" w232 {
              tunnel: w226 -> [_ w265]
              frame False {
                n236 = call "显示对话框信息"() -> ()  [unwired: 10 in, 2 out]
              }
              frame True {
                n237 = Send Notification(notification="DSP" ("通知"), notifier=w265) -> ()  [unwired: 1 in, 2 out]
              }
            }
            n238 = local write "数组_选择"(w227) -> ()
            n239 = Initialize Array(FALSE, 32 ("维数大小"), 5 ("维数大小")) -> (w228:bool[][])
            n240 = local write "合格？"(w228) -> ()
          }
        }
      }
      event "btn_全选": Value Change {
        w267 = TRUE ("单选_AD_1")
        n241 = event-data() -> ()  [unwired: 1 in, 5 out]
        n242 = local write "A_1"(w267) -> ()
        n243 = local write "A_2"(w267) -> ()
        n244 = local write "A_3"(w267) -> ()
        n245 = local write "A_4"(w267) -> ()
        n246 = local write "A_5"(w267) -> ()
        n247 = local write "A_6"(w267) -> ()
        n248 = local write "A_7"(w267) -> ()
        n249 = local write "A_8"(w267) -> ()
        n250 = local write "A_9"(w267) -> ()
        n251 = local write "A_10"(w267) -> ()
        n252 = local write "A_11"(w267) -> ()
        n253 = local write "A_12"(w267) -> ()
        n254 = local write "A_13"(w267) -> ()
        n255 = local write "A_14"(w267) -> ()
        n256 = local write "A_15"(w267) -> ()
        n257 = local write "A_16"(w267) -> ()
        n258 = local write "A_17"(w267) -> ()
        n259 = local write "A_18"(w267) -> ()
        n260 = local write "A_19"(w267) -> ()
        n261 = local write "A_20"(w267) -> ()
        n262 = local write "A_21"(w267) -> ()
        n263 = local write "A_22"(w267) -> ()
        n264 = local write "A_23"(w267) -> ()
        n265 = local write "A_24"(w267) -> ()
        n266 = local write "A_25"(w267) -> ()
        n267 = local write "A_26"(w267) -> ()
        n268 = local write "A_27"(w267) -> ()
        n269 = local write "A_28"(w267) -> ()
        n270 = local write "A_29"(w267) -> ()
        n271 = local write "A_30"(w267) -> ()
        n272 = local write "A_31"(w267) -> ()
        n273 = local write "A_32"(w267) -> ()
      }
      event "btn_反选": Value Change {
        n274 = event-data() -> ()  [unwired: 1 in, 5 out]
        n275 = local read "A_17"() -> (w299:bool)
        n276 = local read "A_18"() -> (w297:bool)
        n277 = local read "A_19"() -> (w295:bool)
        n278 = local read "A_20"() -> (w293:bool)
        n279 = local read "A_21"() -> (w291:bool)
        n280 = local read "A_22"() -> (w289:bool)
        n281 = local read "A_23"() -> (w287:bool)
        n282 = local read "A_24"() -> (w285:bool)
        n283 = local read "A_25"() -> (w283:bool)
        n284 = local read "A_26"() -> (w281:bool)
        n285 = local read "A_27"() -> (w279:bool)
        n286 = local read "A_28"() -> (w277:bool)
        n287 = local read "A_29"() -> (w275:bool)
        n288 = local read "A_30"() -> (w273:bool)
        n289 = local read "A_31"() -> (w271:bool)
        n290 = local read "A_32"() -> (w269:bool)
        n291 = local read "A_1"() -> (w331:bool)
        n292 = local read "A_2"() -> (w329:bool)
        n293 = local read "A_3"() -> (w328:bool)
        n294 = local read "A_4"() -> (w327:bool)
        n295 = local read "A_5"() -> (w326:bool)
        n296 = local read "A_6"() -> (w325:bool)
        n297 = local read "A_7"() -> (w324:bool)
        n298 = local read "A_8"() -> (w323:bool)
        n299 = local read "A_9"() -> (w322:bool)
        n300 = local read "A_10"() -> (w321:bool)
        n301 = local read "A_11"() -> (w320:bool)
        n302 = local read "A_12"() -> (w319:bool)
        n303 = local read "A_13"() -> (w318:bool)
        n304 = local read "A_14"() -> (w317:bool)
        n305 = local read "A_15"() -> (w316:bool)
        n306 = local read "A_16"() -> (w315:bool)
        n307 = Not(x=w331) -> (.not. x?=w330:bool)
        n308 = Not(x=w329) -> (.not. x?=w300:bool)
        n309 = Not(x=w328) -> (.not. x?=w301:bool)
        n310 = Not(x=w327) -> (.not. x?=w302:bool)
        n311 = Not(x=w326) -> (.not. x?=w303:bool)
        n312 = Not(x=w325) -> (.not. x?=w304:bool)
        n313 = Not(x=w324) -> (.not. x?=w305:bool)
        n314 = Not(x=w323) -> (.not. x?=w306:bool)
        n315 = Not(x=w322) -> (.not. x?=w307:bool)
        n316 = Not(x=w321) -> (.not. x?=w308:bool)
        n317 = Not(x=w320) -> (.not. x?=w309:bool)
        n318 = Not(x=w319) -> (.not. x?=w310:bool)
        n319 = Not(x=w318) -> (.not. x?=w311:bool)
        n320 = Not(x=w317) -> (.not. x?=w312:bool)
        n321 = Not(x=w316) -> (.not. x?=w313:bool)
        n322 = Not(x=w315) -> (.not. x?=w314:bool)
        n323 = Not(x=w299) -> (.not. x?=w298:bool)
        n324 = Not(x=w297) -> (.not. x?=w296:bool)
        n325 = Not(x=w295) -> (.not. x?=w294:bool)
        n326 = Not(x=w293) -> (.not. x?=w292:bool)
        n327 = Not(x=w291) -> (.not. x?=w290:bool)
        n328 = Not(x=w289) -> (.not. x?=w288:bool)
        n329 = Not(x=w287) -> (.not. x?=w286:bool)
        n330 = Not(x=w285) -> (.not. x?=w284:bool)
        n331 = Not(x=w283) -> (.not. x?=w282:bool)
        n332 = Not(x=w281) -> (.not. x?=w280:bool)
        n333 = Not(x=w279) -> (.not. x?=w278:bool)
        n334 = Not(x=w277) -> (.not. x?=w276:bool)
        n335 = Not(x=w275) -> (.not. x?=w274:bool)
        n336 = Not(x=w273) -> (.not. x?=w272:bool)
        n337 = Not(x=w271) -> (.not. x?=w270:bool)
        n338 = Not(x=w269) -> (.not. x?=w268:bool)
        n339 = local write "A_1"(w330) -> ()
        n340 = local write "A_2"(w300) -> ()
        n341 = local write "A_3"(w301) -> ()
        n342 = local write "A_4"(w302) -> ()
        n343 = local write "A_5"(w303) -> ()
        n344 = local write "A_6"(w304) -> ()
        n345 = local write "A_7"(w305) -> ()
        n346 = local write "A_8"(w306) -> ()
        n347 = local write "A_9"(w307) -> ()
        n348 = local write "A_10"(w308) -> ()
        n349 = local write "A_11"(w309) -> ()
        n350 = local write "A_12"(w310) -> ()
        n351 = local write "A_13"(w311) -> ()
        n352 = local write "A_14"(w312) -> ()
        n353 = local write "A_15"(w313) -> ()
        n354 = local write "A_16"(w314) -> ()
        n355 = local write "A_17"(w298) -> ()
        n356 = local write "A_18"(w296) -> ()
        n357 = local write "A_19"(w294) -> ()
        n358 = local write "A_20"(w292) -> ()
        n359 = local write "A_21"(w290) -> ()
        n360 = local write "A_22"(w288) -> ()
        n361 = local write "A_23"(w286) -> ()
        n362 = local write "A_24"(w284) -> ()
        n363 = local write "A_25"(w282) -> ()
        n364 = local write "A_26"(w280) -> ()
        n365 = local write "A_27"(w278) -> ()
        n366 = local write "A_28"(w276) -> ()
        n367 = local write "A_29"(w274) -> ()
        n368 = local write "A_30"(w272) -> ()
        n369 = local write "A_31"(w270) -> ()
        n370 = local write "A_32"(w268) -> ()
      }
    }
    n371 = local write "退出？"(w140) -> ()
  }
  n372 = disable-structure shown="禁用" {
    frame Disabled {
      n373 = for {
        N: 32 -> [_]
        i -> [w334]
        n374 = for {
          N: 6 -> [_]
          tunnel: w334 -> [w341]
          i -> [w338]
          n375 = Quotient & Remainder(x=w341, y=2) -> (x-y*floor(x/y)=w339:i32)  [unwired: 1 out]
          n376 = Equal To 0?(x=w339) -> (x = 0?=w342:bool)
          n377 = case shown="假" w342 {
            tunnel: [u32 16448250 u32 15723488] -> w335
            frame False {
            }
            frame True {
            }
          }
          n378 = Bundle(w341, w338) -> (w337:cluster{i32, i32})  [unwired: 1 in]
          n379 = property on="Analog_WC" class="Tbl (严格)"("Active Cell"=w337) -> (error out=w336:errorcluster)  [unwired: 2 in, 1 out]
          n380 = property on="Analog_WC" class="Tbl (严格)"(error in=w336, "Cell BG Color"=w335) -> ()  [unwired: 1 in, 2 out]
        }
      }
    }
    frame Enabled {
    }
  }
  n381 = Obtain Notifier(name (unnamed)=w12, notification data type=w12) -> (notifier out=w14:refnum<notifier>, error out=w13:errorcluster)  [unwired: 2 in, 1 out]
  n382 = Obtain Notifier(name (unnamed)=w2, notification data type=w2) -> (notifier out=w1:refnum<notifier>)  [unwired: 2 in, 2 out]
  n383 = while {
    tunnel: w14 -> [w351]
    tunnel: w13 -> [w350]
    tunnel: [w349] -> w11
    tunnel: [w348] -> w10
    tunnel: w1 -> [w345]
    stop <- w353 stop-if-true
    n384 = Wait Until Next ms Multiple(millisecond multiple=u32 10 ("毫秒倍数")) -> ()  [unwired: 1 out]
    n385 = Wait on Notification(notifier=w351, timeout in ms (-1)=20 ("超时毫秒(-1)"), error in (no error)=w350) -> (notifier out=w349:refnum<notifier>, notification=w355:string, error out=w348:errorcluster)  [unwired: 1 in, 1 out]
    n386 = Equal?(x=w355, y="DSP" ("通知")) -> (x = y?=w346:bool)
    n387 = case shown="真" w346 {
      tunnel: w345 -> [_ w356]
      frame False {
      }
      frame True {
        n388 = stacked-sequence {
          tunnel: w356 -> [w357 _]
          frame #0 {
            n389 = for {
              N: 32 -> [_]
              tunnel: w357 -> [w359]
              i -> [w361]
              n390 = local read "数组_选择"() -> (w362:bool[])
              n391 = local read "数组_设定值"() -> (w363:dbl[][])
              n392 = Index Array(array=w362, index=w361) -> (element=w360:bool)
              n393 = case shown="真" w360 {
                tunnel: w361 -> [_ w365]
                tunnel: w363 -> [_ w367]
                tunnel: w359 -> [_ w364]
                frame False {
                }
                frame True {
                  n394 = disable-structure shown="禁用" {
                    frame Disabled {
                      n395 = call "can开关切换.vi"() -> ()  [unwired: 10 in, 1 out]
                    }
                    frame Enabled {
                    }
                  }
                  n396 = case shown="真" TRUE {
                    tunnel: w365 -> [_ w369]
                    tunnel: w367 -> [_ w370]
                    tunnel: w364 -> [_ w368]
                    frame False {
                    }
                    frame True {
                      n397 = local write "第几组数据"(w369) -> ()
                      n398 = for {
                        N: 5 -> [_]
                        tunnel: w369 -> [w375]
                        tunnel: w370 -> [w374]
                        tunnel: w368 -> [w372]
                        i -> [w373]
                        n399 = while {
                          tunnel: w375 -> [w384]
                          tunnel: w374 -> [w383]
                          tunnel: w373 -> [w382]
                          tunnel: w372 -> [w376]
                          stop <- w379 stop-if-true
                          n400 = local read "同步_1"() -> (w380:i32)
                          n401 = Wait Until Next ms Multiple(millisecond multiple=u32 10 ("毫秒倍数")) -> ()  [unwired: 1 out]
                          n402 = Equal?(x=w380, y=0) -> (x = y?=w381:bool)
                          n403 = case shown="真" w381 {
                            tunnel: w384 -> [_ w390]
                            tunnel: w383 -> [_ w389]
                            tunnel: w382 -> [_ w388]
                            tunnel: [FALSE w387] -> w379
                            tunnel: w376 -> [_ w386]
                            frame False {
                            }
                            frame True {
                              n404 = stacked-sequence {
                                tunnel: w390 -> [w398 _ _]
                                tunnel: w389 -> [w395 _ _]
                                tunnel: w388 -> [w393 _ _]
                                tunnel: [_ _ w409] -> w387
                                tunnel: w386 -> [_ w406 _]
                                frame #0 {
                                # "PCI板卡下发模拟量数据"
                                n405 = global read "试验配置信息.vi" "设定输出通道"() -> (w397:i32[])
                                n406 = To Long Integer(number=w398) -> (32bit integer=w394:i32)
                                n407 = local write "第几个数据"(w393) -> ()
                                n408 = Index Array(array=w395, index (row)=w394, index (col)=w393) -> (element=w391:dbl)
                                n409 = Index Array(array=w397, index=w394) -> (element=w396:i32)
                                n410 = case shown="1" w396 {
                                tunnel: [w402 w405] -> w392
                                tunnel: w391 -> [w400 w403]
                                frame 0, Default {
                                n411 = Build Array(w400, 0.0) -> (w402:dbl[])
                                }
                                frame 1 {
                                n412 = Build Array(0.0, w403) -> (w405:dbl[])
                                }
                                }
                                n413 = call "Convert to Dynamic Data"("Array"=w392) -> ("Dynamic Data Type"=w399:dynamicdata)  [unwired: 3 out]
                                n414 = call "DAQNavi Assistant"("data in(DDT)"=w399) -> ()  [unwired: 2 in, 17 out]
                                }
                                frame #1 {
                                n415 = local write "同步_1"(1 ("y")) -> ()
                                n416 = Send Notification(notification="NumCheck" ("通知"), notifier=w406) -> ()  [unwired: 1 in, 2 out]
                                }
                                frame #2 {
                                n417 = local read "同步_1"() -> (w411:i32)
                                n418 = Equal?(x=w411, y=1) -> (x = y?=w409:bool)
                                }
                              }
                            }
                          }
                        }
                      }
                    }
                  }
                }
              }
            }
          }
          frame #1 {
            n419 = property on="btn_取消" class="Bool"("DisabledEnum"=T1."Enabled" ("禁用")) -> ()  [unwired: 2 in, 2 out]
          }
        }
      }
    }
    n420 = local read "退出？"() -> (w353:bool)
  }
  n421 = Release Notifier(notifier=w11, error in (no error)=w10) -> ()  [unwired: 1 in, 3 out]
  n422 = Obtain Notifier(name (unnamed)=w9, notification data type=w9) -> (notifier out=w8:refnum<notifier>, error out=w7:errorcluster)  [unwired: 2 in, 1 out]
  n423 = while {
    tunnel: w8 -> [w419]
    tunnel: w7 -> [w418]
    tunnel: [w417] -> w6
    tunnel: [w416] -> w5
    stop <- w415 stop-if-true
    n424 = Wait Until Next ms Multiple(millisecond multiple=u32 10 ("毫秒倍数")) -> ()  [unwired: 1 out]
    n425 = Wait on Notification(notifier=w419, timeout in ms (-1)=20 ("超时毫秒(-1)"), error in (no error)=w418) -> (notifier out=w417:refnum<notifier>, notification=w421:string, error out=w416:errorcluster)  [unwired: 1 in, 1 out]
    n426 = Equal?(x=w421, y="NumCheck" ("通知")) -> (x = y?=w413:bool)
    n427 = case shown="真" w413 {
      frame False {
      }
      frame True {
        n428 = call "DAQNavi Assistant2"() -> ("error out"=w426:errorcluster, "data out(DDT)"=w427:dynamicdata)  [unwired: 2 in, 16 out]
        n429 = Unbundle By Name(w426) -> ("status"=w424:bool)
        n430 = case shown="真" w424 {
          frame False {
          }
          frame True {
            n431 = call "超时"() -> ()  [unwired: 10 in, 2 out]
            n432 = local write "同步_1"(0 ("同步_1")) -> ()
          }
        }
        n433 = call "从动态数据转换"("Dynamic Data Type"=w427) -> ("Array"=w428:dbl[])  [unwired: 3 in]
        n434 = To Single Precision Float(number=w428) -> (single precision float=w423:sgl[])
        n435 = Not(x=w424) -> (.not. x?=w425:bool)
        n436 = case shown="真" w425 {
          tunnel: w423 -> [_ w430]
          frame False {
          }
          frame True {
            n437 = stacked-sequence {
              tunnel: w430 -> [w456 _ _ _ _]
              frame #0 {
                n438 = global read "试验配置信息.vi" "设定输入通道"() -> (w455:i32[])
                n439 = local read "第几组数据"() -> (w454:i32)
                n440 = local read "第几组数据"() -> (w441:i32)
                n441 = global read "试验配置信息.vi" "允许误差"() -> (w442:dbl[])
                n442 = global read "试验配置信息.vi" "参数A1"() -> (w450:dbl[])
                n443 = global read "试验配置信息.vi" "参数A2"() -> (w449:dbl[])
                n444 = global read "试验配置信息.vi" "Max"() -> (w443:dbl[])
                n445 = global read "试验配置信息.vi" "min"() -> (w444:dbl[])
                n446 = local read "第几个数据"() -> (w452:i32)
                n447 = local read "数组_设定值"() -> (w466:dbl[][])
                n448 = Index Array(array=w455, index=w454) -> (element=w453:i32)
                n449 = Index Array(array=w456, index=w453) -> (element=w432:sgl)
                n450 = Index Array(array=w443, index=w441) -> (element=w440:dbl)
                n451 = Index Array(array=w444, index=w441) -> (element=w439:dbl)
                n452 = Index Array(array=w450, index=w441) -> (element=w448:dbl)
                n453 = Index Array(array=w449, index=w441) -> (element=w447:dbl)
                n454 = Index Array(array=w442, index=w441) -> (element=w436:dbl)
                n455 = Subtract(x=w440, y=w439) -> (x-y=w438:dbl)
                n456 = local read "Analog_back"() -> (w460:string[][])
                n457 = local read "第几个数据"() -> (w457:i32)
                n458 = Absolute Value(x=w438) -> (abs(x)=w437:dbl)
                n459 = Index Array(array=w466, index (row)=w441, index (col)=w452) -> (element=w451:dbl)
                n460 = local read "数组_选择"() -> (w446:bool[])
                n461 = Number To Fractional String(number=w432, precision (6)=i16 3 ("精度(6)")) -> (F-format string=w431:string)  [unwired: 2 in]
                n462 = call "函数公式.vi"("参数 b"=w447, "参数 a"=w448, "设定值 1"=w451) -> ("y"=w445:dbl)  [unwired: 5 in, 1 out]
                n463 = Replace Array Subset(array=w460, new element=w431, index (row)=w454, index (col)=w457) -> (w459:string[][])
                n464 = call "误差计算.vi"("选择?"=w446, "允许误差"=w436, "模拟量量程范围"=w437, "设定值_1"=w445, "反馈值_1"=w432) -> ("字符串_误差_1"=w434:string, "合格_1?"=w435:bool)  [unwired: 4 in, 1 out]
                n465 = local write "Analog_back"(w459) -> ()
                n466 = local read "第几个数据"() -> (w458:i32)
                n467 = local read "Analog_WC"() -> (w465:string[][])
                n468 = local read "第几组数据"() -> (w463:i32)
                n469 = Replace Array Subset(array=w465, new element=w434, index (row)=w463, index (col)=w458) -> (w464:string[][])
                n470 = local read "合格？"() -> (w461:bool[][])
                n471 = local write "Analog_WC"(w464) -> ()
                n472 = Replace Array Subset(array=w461, new element=w435, index (row)=w463, index (col)=w458) -> (w462:bool[][])
                n473 = local write "合格？"(w462) -> ()
              }
              frame #1 {
                n474 = local read "合格？"() -> (w471:bool[][])
                n475 = local read "第几组数据"() -> (w468:i32)
                n476 = Index Array(array=w471, index (row)=w468) -> (element=w473:bool[])  [unwired: 1 in]
                n477 = And Array Elements(Boolean array=w473) -> (logical AND=w470:bool)
                n478 = local read "数组_选择"() -> (w469:bool[])
                n479 = Index Array(array=w469, index=w468) -> (element=w467:bool)
                n480 = case shown="真" w467 {
                  tunnel: [cluster{u32, u32}[] [{12369084, 12369084}] w476] -> w472
                  tunnel: w470 -> [_ w475]
                  frame False {
                  }
                  frame True {
                    n481 = case shown="真" w475 {
                      tunnel: [cluster{u32, u32}[] [{16730410, 16711680}] cluster{u32, u32}[] [{61205, 6618880}]] -> w476
                      frame False {
                      }
                      frame True {
                      }
                    }
                  }
                }
                n482 = case shown="31" w468 {
                  tunnel: w472 -> [w479 w480 w481 w482 w483 w484 w485 w486 w487 w488 w489 w490 w491 w492 w493 w494 w495 w496 w497 w498 w499 w500 w501 w502 w503 w504 w505 w506 w507 w508 w509 w510]
                  frame 0, Default {
                    n483 = property on="light_1" class="Bool (严格)"("Colors [4]"=w479) -> ()  [unwired: 2 in, 2 out]
                  }
                  frame 1 {
                    n484 = property on="light_2" class="Bool (严格)"("Colors [4]"=w480) -> ()  [unwired: 2 in, 2 out]
                  }
                  frame 2 {
                    n485 = property on="light_3" class="Bool (严格)"("Colors [4]"=w481) -> ()  [unwired: 2 in, 2 out]
                  }
                  frame 3 {
                    n486 = property on="light_4" class="Bool (严格)"("Colors [4]"=w482) -> ()  [unwired: 2 in, 2 out]
                  }
                  frame 4 {
                    n487 = property on="light_5" class="Bool (严格)"("Colors [4]"=w483) -> ()  [unwired: 2 in, 2 out]
                  }
                  frame 5 {
                    n488 = property on="light_6" class="Bool (严格)"("Colors [4]"=w484) -> ()  [unwired: 2 in, 2 out]
                  }
                  frame 6 {
                    n489 = property on="light_7" class="Bool (严格)"("Colors [4]"=w485) -> ()  [unwired: 2 in, 2 out]
                  }
                  frame 7 {
                    n490 = property on="light_8" class="Bool (严格)"("Colors [4]"=w486) -> ()  [unwired: 2 in, 2 out]
                  }
                  frame 8 {
                    n491 = property on="light_9" class="Bool (严格)"("Colors [4]"=w487) -> ()  [unwired: 2 in, 2 out]
                  }
                  frame 9 {
                    n492 = property on="light_10" class="Bool (严格)"("Colors [4]"=w488) -> ()  [unwired: 2 in, 2 out]
                  }
                  frame 10 {
                    n493 = property on="light_11" class="Bool (严格)"("Colors [4]"=w489) -> ()  [unwired: 2 in, 2 out]
                  }
                  frame 11 {
                    n494 = property on="light_12" class="Bool (严格)"("Colors [4]"=w490) -> ()  [unwired: 2 in, 2 out]
                  }
                  frame 12 {
                    n495 = property on="light_13" class="Bool (严格)"("Colors [4]"=w491) -> ()  [unwired: 2 in, 2 out]
                  }
                  frame 13 {
                    n496 = property on="light_14" class="Bool (严格)"("Colors [4]"=w492) -> ()  [unwired: 2 in, 2 out]
                  }
                  frame 14 {
                    n497 = property on="light_15" class="Bool (严格)"("Colors [4]"=w493) -> ()  [unwired: 2 in, 2 out]
                  }
                  frame 15 {
                    n498 = property on="light_16" class="Bool (严格)"("Colors [4]"=w494) -> ()  [unwired: 2 in, 2 out]
                  }
                  frame 16 {
                    n499 = property on="light_17" class="Bool (严格)"("Colors [4]"=w495) -> ()  [unwired: 2 in, 2 out]
                  }
                  frame 17 {
                    n500 = property on="light_18" class="Bool (严格)"("Colors [4]"=w496) -> ()  [unwired: 2 in, 2 out]
                  }
                  frame 18 {
                    n501 = property on="light_19" class="Bool (严格)"("Colors [4]"=w497) -> ()  [unwired: 2 in, 2 out]
                  }
                  frame 19 {
                    n502 = property on="light_20" class="Bool (严格)"("Colors [4]"=w498) -> ()  [unwired: 2 in, 2 out]
                  }
                  frame 20 {
                    n503 = property on="light_21" class="Bool (严格)"("Colors [4]"=w499) -> ()  [unwired: 2 in, 2 out]
                  }
                  frame 21 {
                    n504 = property on="light_22" class="Bool (严格)"("Colors [4]"=w500) -> ()  [unwired: 2 in, 2 out]
                  }
                  frame 22 {
                    n505 = property on="light_23" class="Bool (严格)"("Colors [4]"=w501) -> ()  [unwired: 2 in, 2 out]
                  }
                  frame 23 {
                    n506 = property on="light_24" class="Bool (严格)"("Colors [4]"=w502) -> ()  [unwired: 2 in, 2 out]
                  }
                  frame 24 {
                    n507 = property on="light_25" class="Bool (严格)"("Colors [4]"=w503) -> ()  [unwired: 2 in, 2 out]
                  }
                  frame 25 {
                    n508 = property on="light_26" class="Bool (严格)"("Colors [4]"=w504) -> ()  [unwired: 2 in, 2 out]
                  }
                  frame 26 {
                    n509 = property on="light_27" class="Bool (严格)"("Colors [4]"=w505) -> ()  [unwired: 2 in, 2 out]
                  }
                  frame 27 {
                    n510 = property on="light_28" class="Bool (严格)"("Colors [4]"=w506) -> ()  [unwired: 2 in, 2 out]
                  }
                  frame 28 {
                    n511 = property on="light_29" class="Bool (严格)"("Colors [4]"=w507) -> ()  [unwired: 2 in, 2 out]
                  }
                  frame 29 {
                    n512 = property on="light_30" class="Bool (严格)"("Colors [4]"=w508) -> ()  [unwired: 2 in, 2 out]
                  }
                  frame 30 {
                    n513 = property on="light_31" class="Bool (严格)"("Colors [4]"=w509) -> ()  [unwired: 2 in, 2 out]
                  }
                  frame 31 {
                    n514 = property on="light_32" class="Bool (严格)"("Colors [4]"=w510) -> ()  [unwired: 2 in, 2 out]
                  }
                }
              }
              frame #2 {
                n515 = local read "第几组数据"() -> (w512:i32)
                n516 = local read "第几个数据"() -> (w515:i32)
                n517 = local read "合格？"() -> (w516:bool[][])
                n518 = local read "数组_选择"() -> (w514:bool[])
                n519 = Index Array(array=w516, index (row) #1=w512, index (col) #1=w515, index (col) #2=w515) -> (element #1=w513:bool)  [unwired: 1 in, 1 out]
                n520 = Index Array(array=w514, index=w512) -> (element=w511:bool)
                n521 = case shown="真" w511 {
                  tunnel: w515 -> [_ w520]
                  tunnel: w513 -> [_ w519]
                  tunnel: w512 -> [_ w518]
                  frame False {
                  }
                  frame True {
                    n522 = call "误差表格颜色.vi"("合格？"=w519, "第几组"=w518) -> ("颜色"=w517:u32)  [unwired: 9 in]
                    n523 = Bundle("第几组数据"=w518, "第几个数据"=w520) -> (w522:cluster{"第几组数据":i32, "第几个数据":i32})  [unwired: 1 in]
                    n524 = property on="Analog_WC" class="Tbl (严格)"("Active Cell"=w522) -> (error out=w521:errorcluster)  [unwired: 2 in, 1 out]
                    n525 = property on="Analog_WC" class="Tbl (严格)"(error in=w521, "Cell BG Color"=w517) -> ()  [unwired: 1 in, 2 out]
                  }
                }
              }
              frame #3 {
                n526 = Wait Until Next ms Multiple(millisecond multiple=u32 100 ("毫秒倍数")) -> ()  [unwired: 1 out]
              }
              frame #4 {
                n527 = local write "同步_1"(0 ("同步_1")) -> ()
              }
            }
          }
        }
      }
    }
    n528 = local read "退出？"() -> (w415:bool)
  }
  n529 = Release Notifier(notifier=w6, error in (no error)=w5) -> ()  [unwired: 1 in, 3 out]
